vi "3.2.vi"() -> ()   [LabVIEW 2015]
panel:
  out "最小值":dbl
  out "最大值":dbl
  out "平均值":dbl
  out "波形图":dbl[](graph)
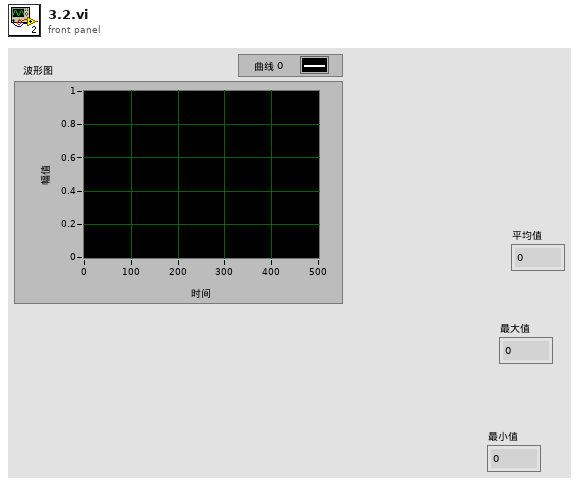
[diagram p1: front panel]
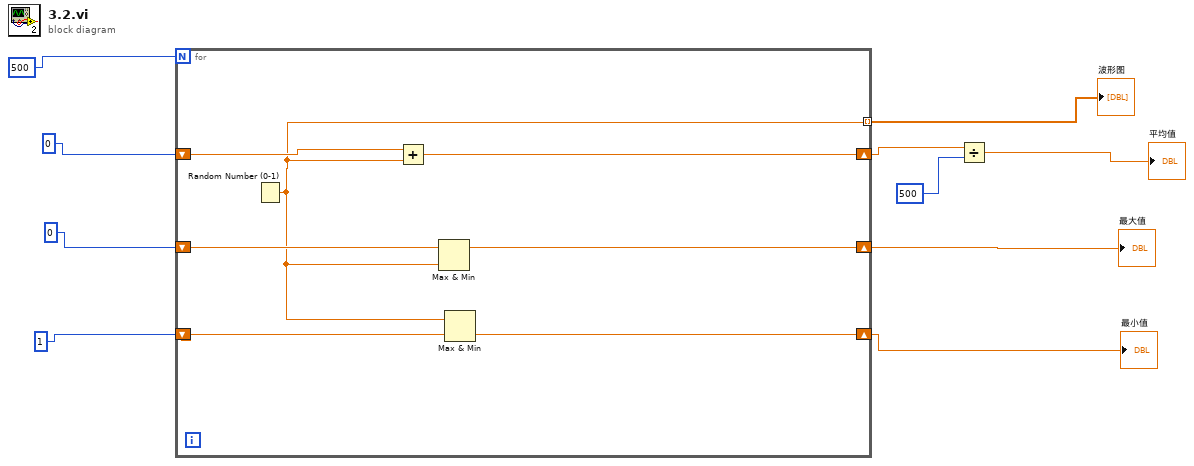
[diagram p0: block diagram]
diagram:
  n1 = for {
    N: 500 -> [_]
    shift-right: [w13] -> w3
    shift-left: 0 -> [w17]
    shift-right: [w12] -> w2
    shift-left: 1 -> [w16]
    shift-right: [w14] -> w4
    shift-left: 0 -> [w15]
    tunnel: [w11] -> w1 mode=indexing
    n2 = Random Number (0-1)() -> (number: 0 to 1=w11:dbl)
    n3 = Add(x=w15, y=w11) -> (x+y=w14:dbl)
    n4 = Max & Min(x=w17, y=w11) -> (max(x,y)=w13:dbl)  [unwired: 1 out]
    n5 = Max & Min(x=w11, y=w16) -> (min(x,y)=w12:dbl)  [unwired: 1 out]
  }
  "波形图" <- w1
  "最小值" <- w2
  "最大值" <- w3
  n6 = Divide(x=w4, y=500) -> (x/y=→"平均值":dbl)
